vi "Convert to Insp, Exp times.vi"(8 "Loop Rate":u16=5, 10 "I:E Ratio":T1=6 max=7 step=1 scale=0.0..7.0, 11 "Brpm":sgl=6.0 format="%#_2g") -> (1 "expcounts":u16, 2 "inspcounts":u16)   [LabVIEW 2016]
uses:
  Controls/IE Ratio knob.ctl
  Miscellaneous/Globals.vi
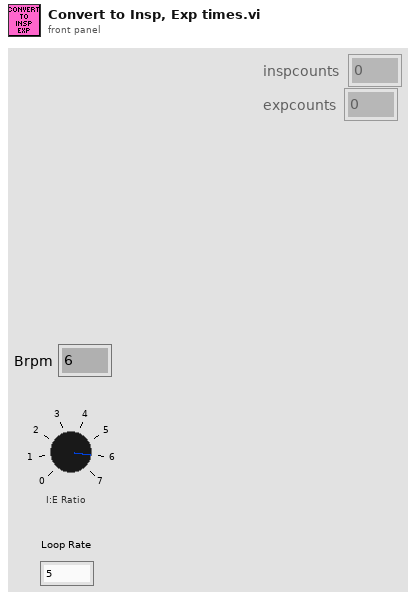
[diagram p1: front panel]
types:
  T1 = typedef "IE Ratio knob.ctl" = u8
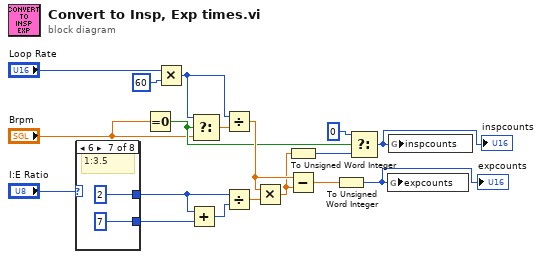
[diagram p0: block diagram]
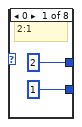
[diagram p2: hidden frame]
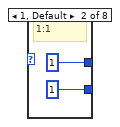
[diagram p3: hidden frame]
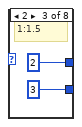
[diagram p4: hidden frame]
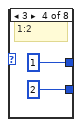
[diagram p5: hidden frame]
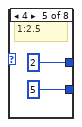
[diagram p6: hidden frame]
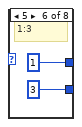
[diagram p7: hidden frame]
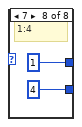
[diagram p8: hidden frame]
diagram:
  n1 = case shown="6" "I:E Ratio" {
    tunnel: [2 1 2 1 2 1 2 1] -> w12
    tunnel: [1 1 3 2 5 3 7 4] -> w11
    frame 0 {
      # "2:1"
    }
    frame 1, Default {
      # "1:1"
    }
    frame 2 {
      # "1:1.5"
    }
    frame 3 {
      # "1:2"
    }
    frame 4 {
      # "1:2.5"
    }
    frame 5 {
      # "1:3"
    }
    frame 6 {
      # "1:3.5"
    }
    frame 7 {
      # "1:4"
    }
  }
  n2 = Equal To 0?(x="Brpm") -> (x = 0?=w9:bool)
  n3 = Multiply(x="Loop Rate", y=u16 60) -> (x*y=w4:u16)
  n4 = Add(x=w12, y=w11) -> (x+y=w18:i32)
  n5 = Select(t=w4, s=w9, f="Brpm") -> (s? t:f=w10:sgl)
  n6 = Divide(x=w4, y=w10) -> (x/y=w16:sgl)
  n7 = Divide(x=w12, y=w18) -> (x/y=w17:dbl)
  n8 = Multiply(x=w16, y=w17) -> (x*y=w15:dbl)
  n9 = To Unsigned Word Integer(number=w15) -> (unsigned 16bit integer=w7:u16)
  n10 = Subtract(x=w16, y=w15) -> (x-y=w14:dbl)
  n11 = To Unsigned Word Integer(number=w14) -> (unsigned 16bit integer=w2:u16)
  "expcounts" <- w2
  n12 = Select(t=0, s=w9, f=w7) -> (s? t:f=w1:i32)
  "inspcounts" <- w1
  n13 = global write "Globals.vi" "expcounts"(w2) -> ()
  n14 = global write "Globals.vi" "inspcounts"(w1) -> ()
